vi "PH_Get6PInformation.get Sixpack Configuration.vi"(5 "error in (no error)":errorcluster) -> (19 "error out":errorcluster)   [LabVIEW 2014, in "PH_Get6PInformation.lvlib"]
doc: "This VI is forseen to to check the axis type depending settings of Sixpack axes."
uses:
  PH_Get6PInformation.lvlib
  PH_Basics/PH_Stepmotor_BaseClass/PH_Stepmotor_BaseClass.Motor Type.ctl
  PH_Devices/PH_Sixpack/PH_Sixpack.Axis Configuration.ctl
  instr.lib/Sixpack/PackDLL/VmaxAmax.ctl
  instr.lib/Sixpack/PackDLL/PeakCurrent.ctl
  instr.lib/Sixpack/PackDLL/VStartVmin.ctl
  instr.lib/Sixpack/PackDLL/Ref Search Parameter.ctl
  instr.lib/Sixpack/PackDLL/Stopswitch Limits.ctl
  instr.lib/Sixpack/PackDLL/Motor Parameter.ctl
  instr.lib/Sixpack/PackDLL/MotorParameter_P5.ctl
  instr.lib/Sixpack/PackDLL/MotorParameter_P6.ctl
  instr.lib/Sixpack/PackDLL/Current Control.ctl
  instr.lib/Sixpack/PackDLL/Current.ctl
  PH_Basics/PH_Stepmotor_BaseClass/PH_Stepmotor_BaseClass.lvlib
  PH_Devices/PH_Sixpack/PH_Sixpack.lvlib
  instr.lib/Sixpack/Sixpack - Driver.lvlib
panel:
  out "6P Axis Config":T1={"VmaxAmax"={"VMax(511)"=511, "AMax(128)"=128}, "I max (50%)"=50.0, "VStartVminDivi"={"VStart(5)"=5, "Vmin(4)"=4, "Div i (2)"=enum."2"}, "Ref Search Parameter"={"VRefMax(100)"=100, "DebouncingTime (22ms)"=34}, "Stopswitch Limits"={"MinLeft(0)"=0, "MaxRight(1023)"=1023}, "Axis Parameter"={"Poslimit (6400)"=6400, "P5 Bits"={"MT_PI"=FALSE, "MT_ROTARY"=FALSE, "MT_AUTONULLCMD"=FALSE, "MT_TESTNULL"=FALSE, "MT_NULLLEFT"=FALSE, "MT_NULLCENTRE"=TRUE, "MT_STOPNULL"=FALSE, "MT_FILTERSWITCH"=TRUE}, "P6 Bits"={"MT_OPTIMIZEWAY"=FALSE, "MT_FASTREF"=TRUE, "MT_MECHREF"=FALSE, "MT_DELAYTESTNULL"=TRUE, "MT_STOPSOFT"=FALSE, "MT_STOPNOREF"=FALSE, "MT_NULLPOSITIVE"=FALSE, "MUT_STOPFULSTEPS"=FALSE}}, "I Control"={"PowerDownDelay (500)"=500, "PowerDown (0%)"=enum."0%", "Standing (50%)"=enum."50%", "Running (75%)"=enum."75%", "Accelerating (100%)"=enum."100%"}} {"Axis Parameter"."Poslimit (6400)" step=1; "Ref Search Parameter"."DebouncingTime (22ms)" format="%.0x"; "I max (50%)" min=0.0 max=100.0}
  in  "Delete":bool
  in  "Motor Type":T12
  # "PCS"
  # "3.40"
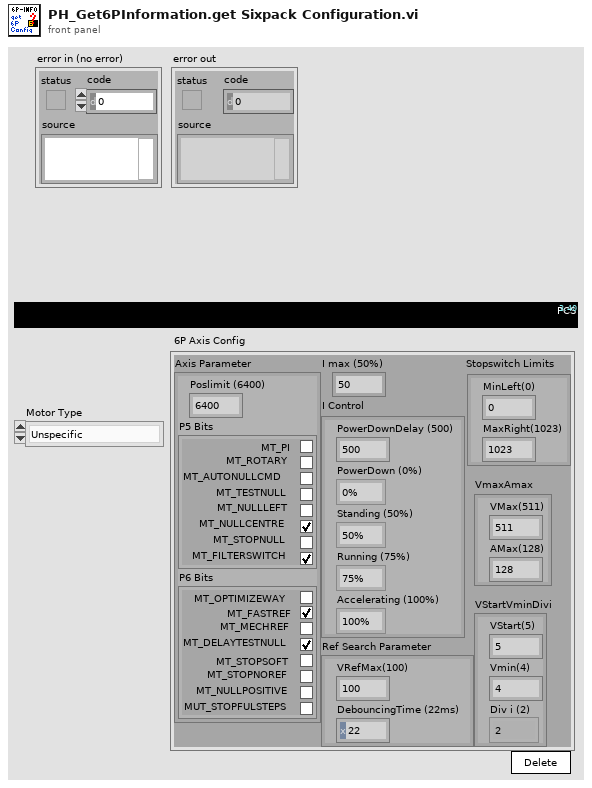
[diagram p1: front panel]
types:
  T1 = typedef "PH_Sixpack.lvlib/PH_Sixpack.Axis Configuration.ctl" = cluster{"VmaxAmax":T2, "I max (50%)":T3, "VStartVminDivi":T4, "Ref Search Parameter":T5, "Stopswitch Limits":T6, "Axis Parameter":T7, "I Control":T10}
  T2 = typedef "Sixpack - Driver.lvlib/VmaxAmax.ctl" = cluster{"VMax(511)":u16, "AMax(128)":u16}
  T3 = typedef "Sixpack - Driver.lvlib/PeakCurrent.ctl" = dbl
  T4 = typedef "Sixpack - Driver.lvlib/VStartVmin.ctl" = cluster{"VStart(5)":u16, "Vmin(4)":u16, "Div i (2)":enum8{"0", "1", "2", "3"}}
  T5 = typedef "Sixpack - Driver.lvlib/Ref Search Parameter.ctl" = cluster{"VRefMax(100)":u16, "DebouncingTime (22ms)":u8}
  T6 = typedef "Sixpack - Driver.lvlib/Stopswitch Limits.ctl" = cluster{"MinLeft(0)":u16, "MaxRight(1023)":u16}
  T7 = typedef "Sixpack - Driver.lvlib/Motor Parameter.ctl" = cluster{"Poslimit (6400)":u32, "P5 Bits":T8, "P6 Bits":T9}
  T8 = typedef "Sixpack - Driver.lvlib/MotorParameter_P5.ctl" = cluster{"MT_PI":bool, "MT_ROTARY":bool, "MT_AUTONULLCMD":bool, "MT_TESTNULL":bool, "MT_NULLLEFT":bool, "MT_NULLCENTRE":bool, "MT_STOPNULL":bool, "MT_FILTERSWITCH":bool}
  T9 = typedef "Sixpack - Driver.lvlib/MotorParameter_P6.ctl" = cluster{"MT_OPTIMIZEWAY":bool, "MT_FASTREF":bool, "MT_MECHREF":bool, "MT_DELAYTESTNULL":bool, "MT_STOPSOFT":bool, "MT_STOPNOREF":bool, "MT_NULLPOSITIVE":bool, "MUT_STOPFULSTEPS":bool}
  T10 = typedef "Sixpack - Driver.lvlib/Current Control.ctl" = cluster{"PowerDownDelay (500)":u16, "PowerDown (0%)":T11, "Standing (50%)":T11, "Running (75%)":T11, "Accelerating (100%)":T11}
  T11 = typedef "Sixpack - Driver.lvlib/Current.ctl" = enum8{"100%", "75%", "50%", "38%", "25%", "19%", "13%", "9%", "0%"}
  T12 = typedef "PH_Stepmotor_BaseClass.lvlib/PH_Stepmotor_BaseClass.Motor Type.ctl" = enum16{"Unspecific", "OWIS 49.120.2633", "OWIS 49.060.1033", "OWIS 43.040.2558", "Diamond Motion 2200 series", "OWIS 49.120.266B.MV6", "Calorimeter", "Linear Stage 1", "MICOS VT-80", "MICOS VT-80 S", "Standa Rotstage nt0.95A", "PUF RA 320.200", "PUF RA 800.200", "PUF RA 800.400", "PUF RA 400.50", "1324.nn.800.50", "1324.n9c.800.50", "1324.nn.320.200", "1324.nn.400.200", "1324.nn.800.200", "1324.nn.400.50", "1324.8c9c.800.50", "1324.8c9c.400.200"}
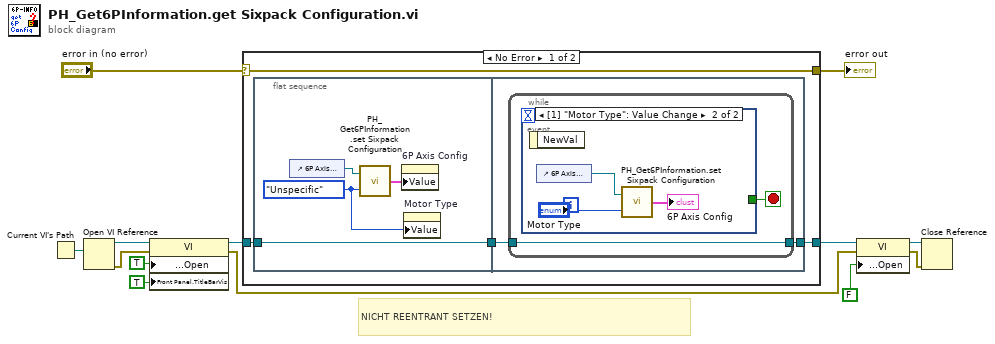
[diagram p0: block diagram]
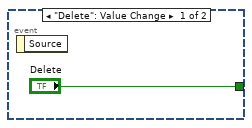
[diagram p2: hidden frame]
diagram:
  # "NICHT REENTRANT SETZEN!"
  n1 = Current VI's Path() -> (path=w11:path)
  n2 = Open VI Reference(vi path=w11) -> (vi reference=w1:refnum<vi>, error out=w5:errorcluster)  [unwired: 5 in]
  n3 = property class="VI"(reference=w1, error in=w5, "Front Panel Window:Open"=TRUE, "Front Panel.TitleBarVis"=TRUE ("Front Panel Window:Title Bar Visible")) -> (reference out=w9:refnum<vi>, error out=w4:errorcluster)
  n4 = case shown="No Error" "error in (no error)" {
    selector: "error in (no error)" -> [w17 w31]
    tunnel: [w17 w31] -> w13
    tunnel: w9 -> [w16 w30]
    tunnel: [w15 w30] -> w7
    frame No Error {
      n5 = flat-sequence {
        tunnel: w16 -> [w21]
        tunnel: [w21] -> w14
        tunnel: [w22] -> w15
        tunnel: w14 -> [w23]
        frame #0 {
          w20 = PH_Stepmotor_BaseClass.Motor_Type."Unspecific" ("Motor Type")
          n6 = control-ref of="6P Axis Config"() -> (w18:refnum<vi>)
          n7 = call "PH_Get6PInformation.set Sixpack Configuration.vi"("Motor Type"=w20, "6P Axis Config Ref"=w18) -> ("6P Axis Config"=w19:T1)
          n8 = property on="6P Axis Config" class="Clust (strict)"("Value"=w19) -> ()  [unwired: 2 in, 2 out]
          n9 = property on="Motor Type" class="Enum (strict)"("Value"=w20) -> ()  [unwired: 2 in, 2 out]
        }
        frame #1 {
          n10 = while {
            tunnel: w23 -> [w25]
            tunnel: [w25] -> w22
            stop <- w24 stop-if-true
            n11 = event shown="[1] \"Motor Type\": Value Change" {
              selector: _ -> [_ _]
              dyn-events: _ -> [_ _]
              timeout: _ -> [_ _]
              tunnel: ["Delete" _] -> w24
              event "Delete": Value Change {
                n12 = event-data() -> ()  [unwired: 1 in, 1 out]
              }
              event Value Change {
                n13 = event-data() -> ()  [unwired: 1 in, 1 out]
                n14 = control-ref of="6P Axis Config"() -> (w28:refnum<vi>)
                n15 = call "PH_Get6PInformation.set Sixpack Configuration.vi"("Motor Type"="Motor Type", "6P Axis Config Ref"=w28) -> ("6P Axis Config"=→"6P Axis Config":T1)
              }
            }
          }
        }
      }
    }
    frame Error {
    }
  }
  "error out" <- w13
  n16 = property class="VI"(reference=w7, error in=w4, "Front Panel Window:Open"=FALSE) -> (reference out=w6:refnum<vi>, error out=w3:errorcluster)
  n17 = Close Reference(reference=w6, error in (no error)=w3) -> ()  [unwired: 1 out]
